vi "Force_rewrite_permissions.vi"(8 "error in (no error)":errorcluster, 10 "Desktop Path":path, 11 "Waveforms Path":path) -> (0 "error out":errorcluster)   [LabVIEW 2013]
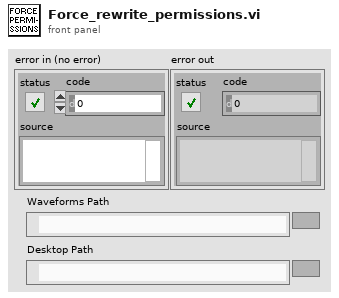
[diagram p1: front panel]
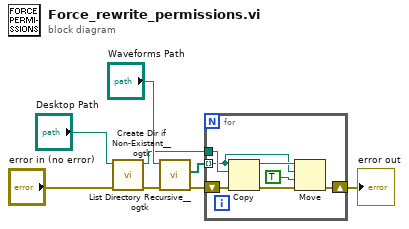
[diagram p0: block diagram]
diagram:
  n1 = call <userlib>:"Create Dir if Non-Existant__ogtk.vi"("error in (no error)"="error in (no error)", "Directory Path"="Desktop Path") -> ("error out"=w7:errorcluster, "dup Directory Path"=w4:path)  [unwired: 7 in, 1 out]
  n2 = call <userlib>:"List Directory Recursive__ogtk.vi"("error in (no error)"=w7, "Path"="Waveforms Path") -> ("error out"=w5:errorcluster, "file paths"=w1:path[])  [unwired: 6 in, 2 out]
  n3 = for {
    shift-right: [w12] -> w3
    shift-left: w5 -> [w15]
    tunnel: w4 -> [w10]
    tunnel: w1 -> [w9] mode=indexing
    n4 = Copy(8:w15, 10:w10, 11:w9) -> (0:w13:errorcluster, 3:w11:path)  [unwired: 2 in, 1 out]
    n5 = Move(source path=w11, error in=w13, 9:TRUE ("overwrite (F)"), 10:w9) -> (error out=w12:errorcluster)  [unwired: 1 in, 2 out]
  }
  "error out" <- w3
